vi "Initialize Kalman Filter.vi"(8 "Dynamical System Matrices":T3, 9 "Initial Control Input":T2, 10 "Guessed Initial Covariance":T2, 11 "Guessed Initial State":T2) -> (3 "Kalman Filter":T1)   [LabVIEW 2020]
uses:
  ctl/Dynamical System Matrices.ctl
  <vilib>/Analysis/Matrix/Datatypes/RealMatrix.ctl
  ctl/Kalman Filter Instance.ctl
  <vilib>/Analysis/Matrix/NI_Matrix.lvlib
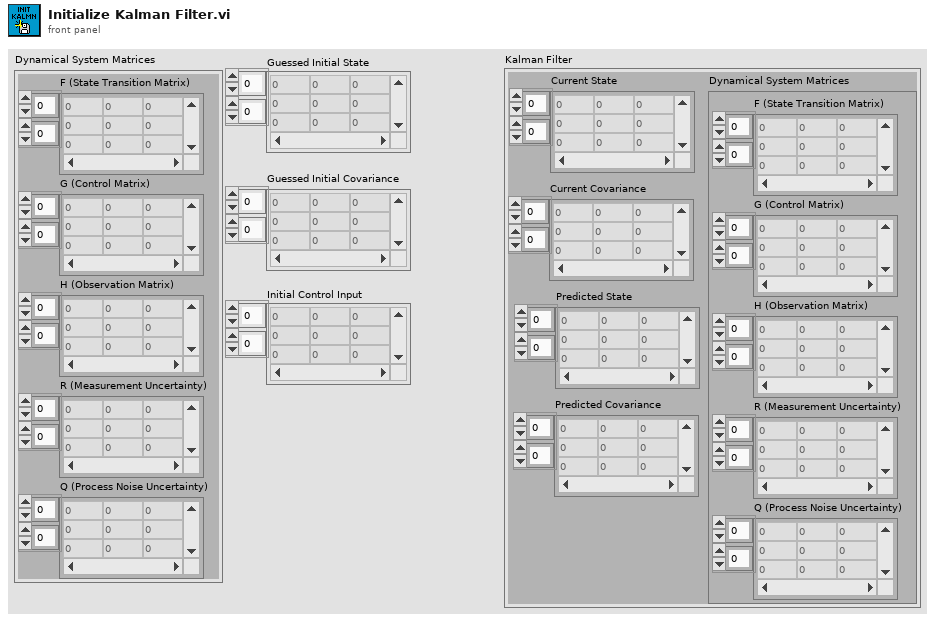
[diagram p1: front panel]
types:
  T1 = typedef "Kalman Filter Instance.ctl" = cluster{"Current State":T2, "Current Covariance":T2, "Predicted State":T2, "Predicted Covariance":T2, "Dynamical System Matrices":T3}
  T2 = typedef "NI_Matrix.lvlib/RealMatrix.ctl" = dbl[][]
  T3 = typedef "Dynamical System Matrices.ctl" = cluster{"F (State Transition Matrix)":T2, "G (Control Matrix)":T2, "H (Observation Matrix)":T2, "R (Measurement Uncertainty)":T2, "Q (Process Noise Uncertainty)":T2}
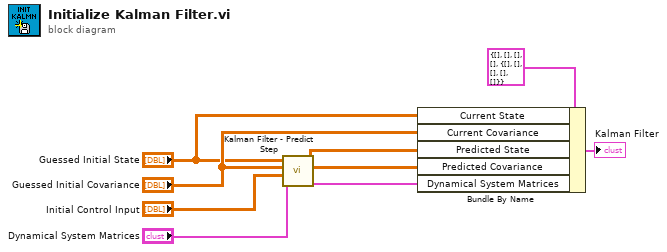
[diagram p0: block diagram]
diagram:
  n1 = call "Kalman Filter - Predict Step.vi"("Dynamical System Matrices In"="Dynamical System Matrices", "Control Input"="Initial Control Input", "Initial Covariance"="Guessed Initial Covariance", "Initial State"="Guessed Initial State") -> ("Dynamical System Matrices Out"=w5:T3, "Predicted Covariance"=w4:T2, "Predicted State"=w6:T2)  [unwired: 5 in]
  n2 = Bundle By Name(cluster=T1 {"Current State"=[], "Current Covariance"=[], "Predicted State"=[], "Predicted Covariance"=[], "Dynamical System Matrices"={"F (State Transition Matrix)"=[], "G (Control Matrix)"=[], "H (Observation Matrix)"=[], "R (Measurement Uncertainty)"=[], "Q (Process Noise Uncertainty)"=[]}} ("Kalman Filter In 2"), "Current State"="Guessed Initial State", "Current Covariance"="Guessed Initial Covariance", "Predicted State"=w6, "Predicted Covariance"=w4, "Dynamical System Matrices"=w5) -> (→"Kalman Filter":T1)
